vi "Measure Sound from Reference Mic.vi"() -> ()   [LabVIEW 2022 SP3]
doc: "Overview:\nThis VI demonstrates sound pressure acquisition with an IEPE microphone and fractional-octave analysis with running sound level measurements.\n\nRequirements:\nLabVIEW Full Development System\nSound and Vibration Toolkit\n\nInstructions:\n1. Select the DAQmx physical channel connected to microphone.\n2. Run the VI.\n\nDetails:\nThis VI continuously acquires sound pressure data from the specified channel. This VI then applies the specified weighting filter, computes a third-octave spectrum, and measures the equivalent continuous level (Leq) and a decimated exponential average level.\n\nThis VI is suitable to run on a real-time (RT) target."
uses:
  <vilib>/DAQmx/read.llb/DAQmx Read (Analog Wfm 1Chan NSamp).vi
  <vilib>/DAQmx/create/channels.llb/DAQmx Create Channel (AI-Sound Pressure-Microphone).vi
  <vilib>/DAQmx/configure/timing.llb/DAQmx Timing (Sample Clock).vi
  <vilib>/DAQmx/miscellaneous.llb/DAQmx Fill In Error Info.vi
  <vilib>/addons/Sound and Vibration/svt_Weighting/SVT Weighting Filter (1 Ch).vi
  <vilib>/addons/Sound and Vibration/svt_Level/SVL Leq Sound Level (1 Ch).vi
  <vilib>/addons/Sound and Vibration/svt_Weighting/SoundVib_ABCWeighting.lvlib
  <vilib>/addons/Sound and Vibration/svt_Level/SoundVib_SoundLevel.lvlib
panel:
  out "Leq sound level [dB EU]":dbl=69.10880378464721 format="%.2f"
  out "Waveform Graph":waveform(dbl)(graph)={"t0"=timestamp(3812036814.2232547 s since 1904-01-01), "dt"=1.9999999995925458e-05, "Y"=array[5000 elements], "attributes"=variant("NI_ChannelName"=variant(string "PXI1Slot2/ai0"), "NI_UnitDescription"=variant(string "Pascals"), "NI_dBReference"=variant(dbl 2e-05))}
  in  "sensor sensitivity [mV/Pa]":dbl=50.0
  in  "physical channel":tag="PXI1Slot2/ai0"
  in  "weighting":u16(ring) items=["Linear", "A-weighting", "B-weighting", "C-weighting"]
  in  "quit":bool
  # "Channel Settings"
  # "Analysis Settings"
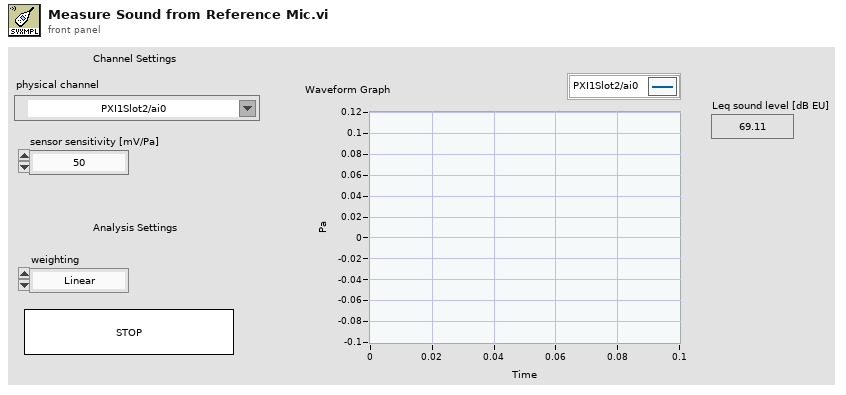
[diagram p1: front panel]
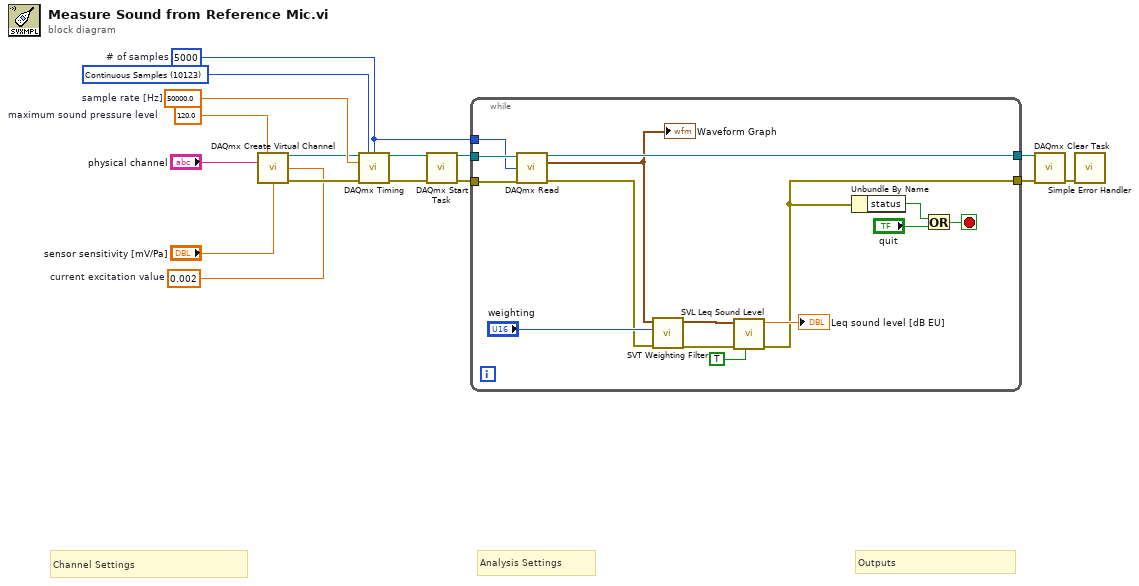
[diagram p0: block diagram]
diagram:
  w2 = 0.002  # current excitation value
  w5 = 5000  # # of samples
  w10 = 50000.0  # sample rate [Hz]
  w7 = 120.0  # maximum sound pressure level
  w16 = 10123 items=["Finite Samples"=10178, "Continuous Samples"=10123] ("sample mode")
  # "Outputs"
  # "Analysis Settings"
  # "Channel Settings"
  n1 = call-poly <vilib>:"DAQmx Create Virtual Channel.vi"("maximum sound pressure level"=w7, "physical channels"="physical channel", "current excitation value"=w2, "microphone sensitivity"="sensor sensitivity [mV/Pa]") -> ("task out"=w4:refnum<k21>, "error out"=w3:errorcluster)  [unwired: 10 in]
  n2 = call-poly <vilib>:"DAQmx Timing.vi"("task/channels in"=w4, "sample mode"=w16, "samples per channel"=w5, "rate"=w10, "error in"=w3) -> ("task out"=w15:refnum<k21>, "error out"=w12:errorcluster)  [unwired: 9 in]
  n3 = call <vilib>:"DAQmx Start Task.vi"("task/channels in"=w15, "error in"=w12) -> ("task out"=w14:refnum<k21>, "error out"=w13:errorcluster)  [unwired: 12 in]
  n4 = while {
    tunnel: [w18] -> w8
    tunnel: [w26] -> w9
    tunnel: w13 -> [w28]
    tunnel: w14 -> [w29]
    tunnel: w5 -> [w22]
    stop <- w30 stop-if-true
    n5 = call-poly <vilib>:"DAQmx Read.vi"("task/channels in"=w29, "number of samples per channel"=w22, "error in"=w28) -> ("task out"=w26:refnum<k21>, "data"=w20:waveform(dbl), "error out"=w23:errorcluster)  [unwired: 10 in]
    "Waveform Graph" <- w20
    n6 = call-poly <vilib>:"SVT Weighting Filter.vi"("error in (no error)"=w23, "weighting"="weighting", "scaled signal [EU]"=w20) -> ("error out"=w24:errorcluster, "weighted signal [EU]"=w25:waveform(dbl))  [unwired: 6 in]
    n7 = call-poly <vilib>:"SVL Leq Sound Level.vi"("restart averaging (F)"=TRUE, "error in (no error)"=w24, "scaled signal [EU]"=w25) -> ("error out"=w18:errorcluster, "Leq sound level [dB EU]"=→"Leq sound level [dB EU]":dbl)  [unwired: 6 in, 1 out]
    n8 = Unbundle By Name(w18) -> ("status"=w21:bool)
    n9 = Or(x=w21, y="quit") -> (x .or. y?=w30:bool)
  }
  n10 = call <vilib>:"DAQmx Clear Task.vi"("task in"=w9, "error in"=w8) -> ("error out"=w1:errorcluster)  [unwired: 13 in]
  n11 = call <vilib>:"Simple Error Handler.vi"("error in (no error)"=w1) -> ()  [unwired: 4 in, 5 out]
